vi "Set guard and sense.vi"(8 "error in":errorcluster, 9 "Sense (Unchanged)":u16(ring)=2 items=["Local", "Remote", "Unchanged"], 10 "Guard (Unchanged)":u16(ring)=2 items=["Local", "Remote", "Unchanged"], 11 "VISA resource name":refnum<visa-resource-name>) -> (0 "error out":errorcluster, 1 "Remote sense?":i32, 2 "Remote guard?":i32, 3 "VISA resource name out":refnum<visa-resource-name>)   [LabVIEW 2020, in "Datron D4xxx.lvlib"]
doc: "This VI sets guard and sense modes. If you select \"Unchanged\", VI just returns current state."
uses:
  Datron D4xxx.lvlib
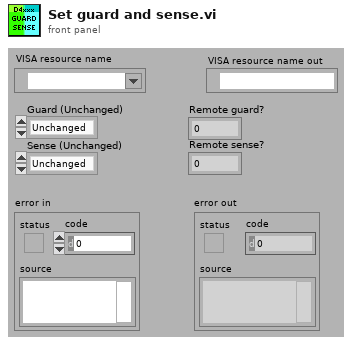
[diagram p1: front panel]
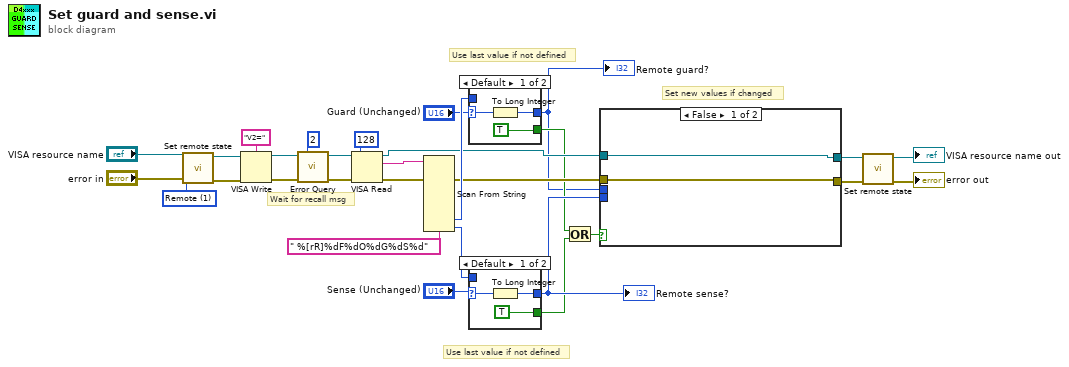
[diagram p0: block diagram]
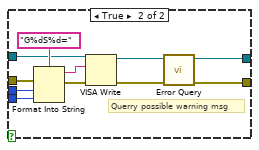
[diagram p2: hidden frame]
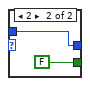
[diagram p3: hidden frame]
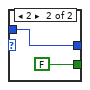
[diagram p4: hidden frame]
diagram:
  w26 = u16 1 items=["Local", "Remote", "Default"] ("Remote state")
  # "Use last value if not defined"
  # "Use last value if not defined"
  # "Set new values if changed"
  # "Wait for recall msg"
  n1 = call "Set remote state.vi"("error in"="error in", "Remote state"=w26, "VISA resource name"="VISA resource name") -> ("error out"=w13:errorcluster, "VISA resource name out"=w12:refnum<visa-resource-name>)  [unwired: 7 in]
  n2 = VISA Write(VISA resource name=w12, write buffer="V2=", error in (no error)=w13) -> (VISA resource name out=w15:refnum<visa-resource-name>, error out=w16:errorcluster)  [unwired: 1 out]
  n3 = call "Error Query.vi"("error in (no error)"=w16, "Check cycles (11)"=2, "VISA resource name"=w15) -> ("error out"=w18:errorcluster, "VISA resource name out"=w17:refnum<visa-resource-name>)  [unwired: 5 in, 2 out]
  n4 = VISA Read(VISA resource name=w17, byte count=u32 128, error in (no error)=w18) -> (VISA resource name out=w5:refnum<visa-resource-name>, read buffer=w19:string, error out=w21:errorcluster)  [unwired: 1 out]
  n5 = Scan From String(format string=" %[rR]%dF%dO%dG%dS%d", input string=w19, error in=w21) -> (error out=w6:errorcluster, output 5=w9:i32, output 6=w10:i32)  [unwired: 11 in, 2 out]
  n6 = case shown="Default" "Guard (Unchanged)" {
    selector: "Guard (Unchanged)" -> [w33 _]
    tunnel: [w32 w35] -> w1
    tunnel: w9 -> [_ w35]
    tunnel: [TRUE FALSE] -> w3
    frame Default {
      n7 = To Long Integer(number=w33) -> (32bit integer=w32:i32)
    }
    frame 2 {
    }
  }
  "Remote guard?" <- w1
  n8 = case shown="Default" "Sense (Unchanged)" {
    selector: "Sense (Unchanged)" -> [w38 _]
    tunnel: w10 -> [_ w40]
    tunnel: [w37 w40] -> w7
    tunnel: [TRUE FALSE] -> w2
    frame Default {
      n9 = To Long Integer(number=w38) -> (32bit integer=w37:i32)
    }
    frame 2 {
    }
  }
  "Remote sense?" <- w7
  n10 = Or(x=w3, y=w2) -> (x .or. y?=w4:bool)
  n11 = case shown="False" w4 {
    tunnel: [w42 w49] -> w25
    tunnel: [w41 w47] -> w24
    tunnel: w1 -> [_ w46]
    tunnel: w7 -> [_ w45]
    tunnel: w6 -> [w42 w44]
    tunnel: w5 -> [w41 w43]
    frame False {
    }
    frame True {
      # "Querry possible warning msg"
      n12 = Format Into String(format string="G%dS%d=", error in=w44, w46, w45) -> (resulting string=w53:string, error out=w52:errorcluster)  [unwired: 1 in]
      n13 = VISA Write(VISA resource name=w43, write buffer=w53, error in (no error)=w52) -> (VISA resource name out=w48:refnum<visa-resource-name>, error out=w50:errorcluster)  [unwired: 1 out]
      n14 = call "Error Query.vi"("error in (no error)"=w50, "VISA resource name"=w48) -> ("error out"=w49:errorcluster, "VISA resource name out"=w47:refnum<visa-resource-name>)  [unwired: 6 in, 2 out]
    }
  }
  n15 = call "Set remote state.vi"("error in"=w25, "VISA resource name"=w24) -> ("error out"=→"error out":errorcluster, "VISA resource name out"=→"VISA resource name out":refnum<visa-resource-name>)  [unwired: 8 in]
